vi "Update State.vi"(8 "error in (no error)":errorcluster, 11 "Elevator Controller in":refnum<class "Elevator Controller.lvclass">) -> (0 "error out":errorcluster, 3 "Elevator Controller out":refnum<class "Elevator Controller.lvclass">)   [LabVIEW 2022 SP3, in "Elevator Controller.lvlib" / "Elevator Controller.lvclass"]
uses:
  Elevator Controller.lvclass
  Sim User Console Actor/Abstract User Console Actor/Sim User Console Actor.lvclass
  Abstract User Console Actor/Abstract User Console Actor/Elevator Call.ctl
  Abstract User Console Actor/Abstract User Console Actor/Abstract User Console Actor.lvclass
  Abstract User Console Actor/Abstract User Console Actor/Floor Selection.ctl
  Sim Display Console Actor/Sim Display Console Actor/Sim Display Console Actor.lvclass
  Sim Sensor Interface Actor/Sim Sensor Interface Actor/Sim Sensor Interface Actor.lvclass
  States -Enum.ctl
  Configuration Database Actor/Configuration Database Actor/Configuration Database Actor.lvclass
  <vilib>/ActorFramework/Actor/Actor.lvclass
  Incoming Messages/Set State Msg/Set State Msg.lvclass
  C:/Program Files/National Instruments/LabVIEW 2022/vi.lib/ActorFramework/Actor/Actor.lvclass
  C:/Workspace/CLA/Elevator AF_2022/Elevator Controller/Elevator Controller/Elevator Controller.lvclass
  C:/Workspace/CLA/Elevator AF_2022/Incoming/Incoming.lvclass
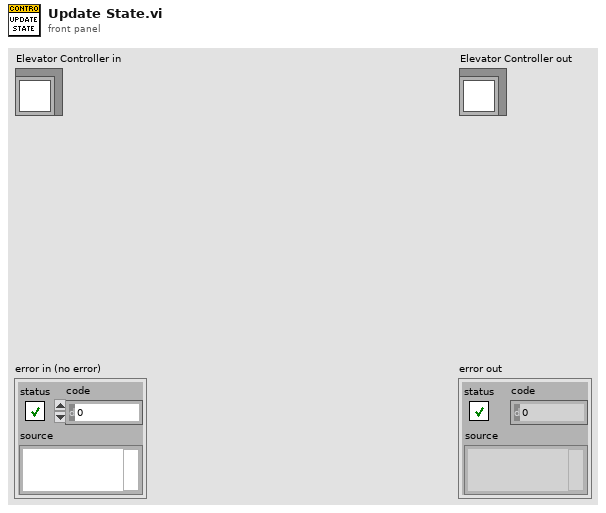
[diagram p1: front panel]
types:
  T1 = typedef "Abstract User Console Actor.lvlib/Abstract User Console Actor.lvclass/Floor Selection.ctl" = cluster{"Floor4":bool, "Floor 3":bool, "Floor2":bool, "Floor1":bool}
  T2 = typedef "Abstract User Console Actor.lvlib/Abstract User Console Actor.lvclass/Elevator Call.ctl" = cluster{"Up":bool, "Up 2":bool, "Up 3":bool, "Down":bool, "Down 2":bool, "Down 3":bool}
  T3 = typedef "Elevator Controller.lvlib/Elevator Controller.lvclass/States -Enum.ctl" = enum16{"Initial State", "Wait for First Request", "Start and Move State", "Analysis State", "Continue Travel State", "Stop at Floor", "Open and Close Door Sequence", "No Request Remaining", "Emergency Call", "Terminate Process", ""}
  T4 = enum8{"Enabled", "Disabled", "Disabled and Grayed Out"}
  T5 = typedef "Configuration Database Actor.lvlib/Configuration Database Actor.lvclass/Time Table.ctl" = cluster{"Open Door":u32, "Close Door":u32, "Travel Time":u32, "Inactivity Time":u32}
  T6 = typedef "Abstract User Console Actor.lvlib/Abstract User Console Actor.lvclass/Door Buttons.ctl" = cluster{"Open Door":bool, "Close Door":bool}
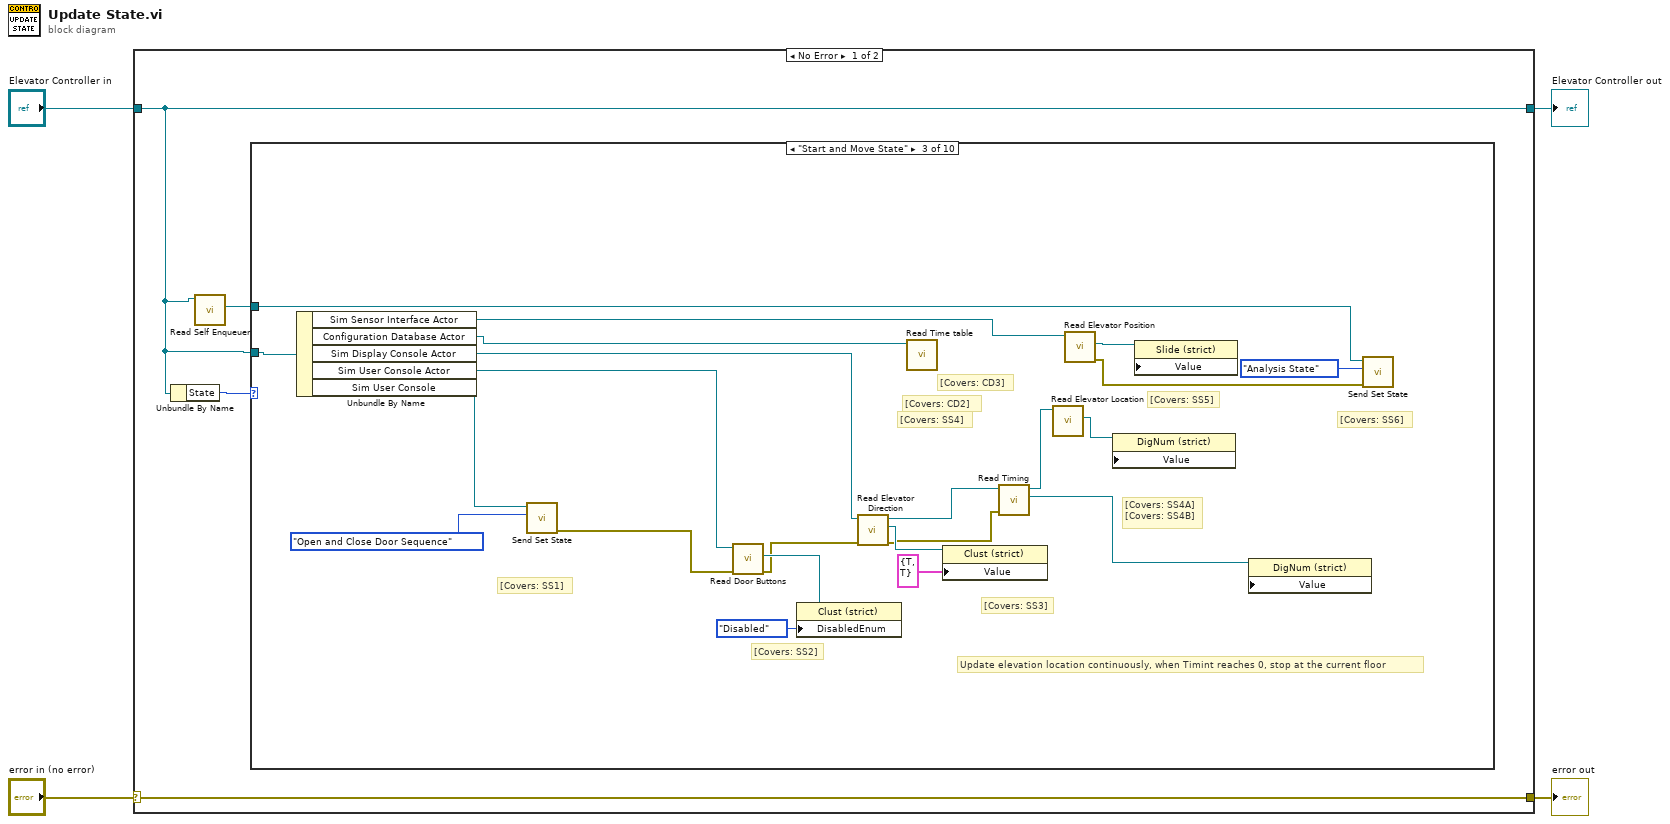
[diagram p0: block diagram]
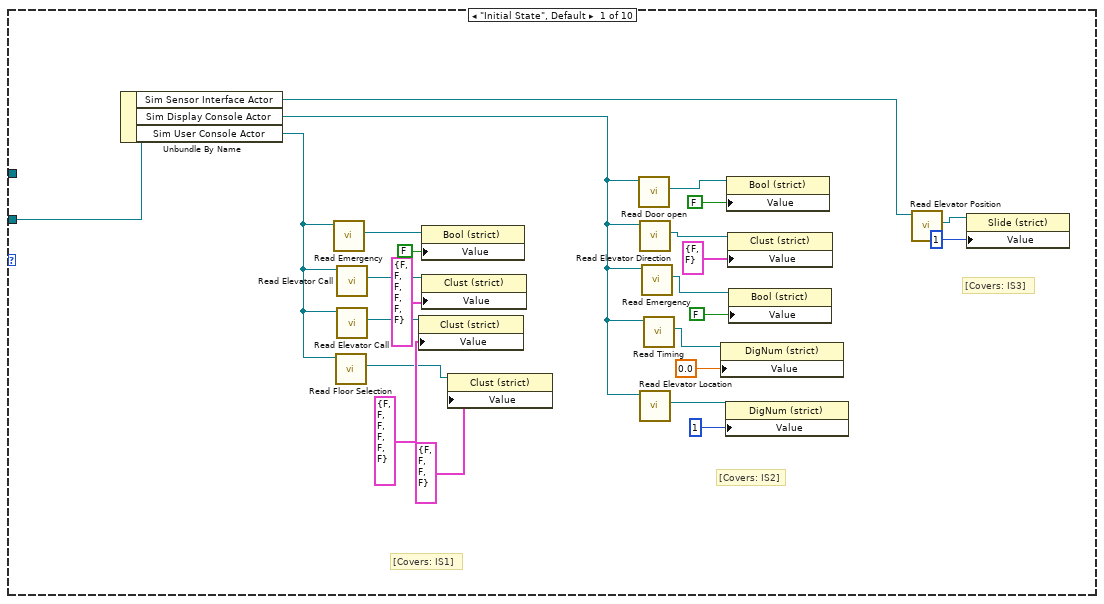
[diagram p2: hidden frame]
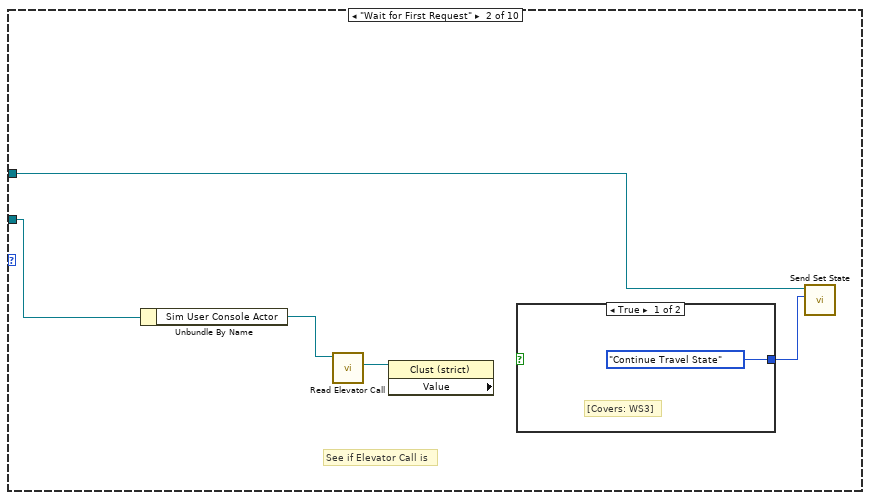
[diagram p3: hidden frame]
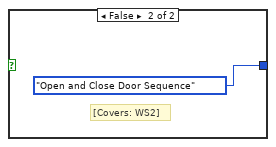
[diagram p4: hidden frame]
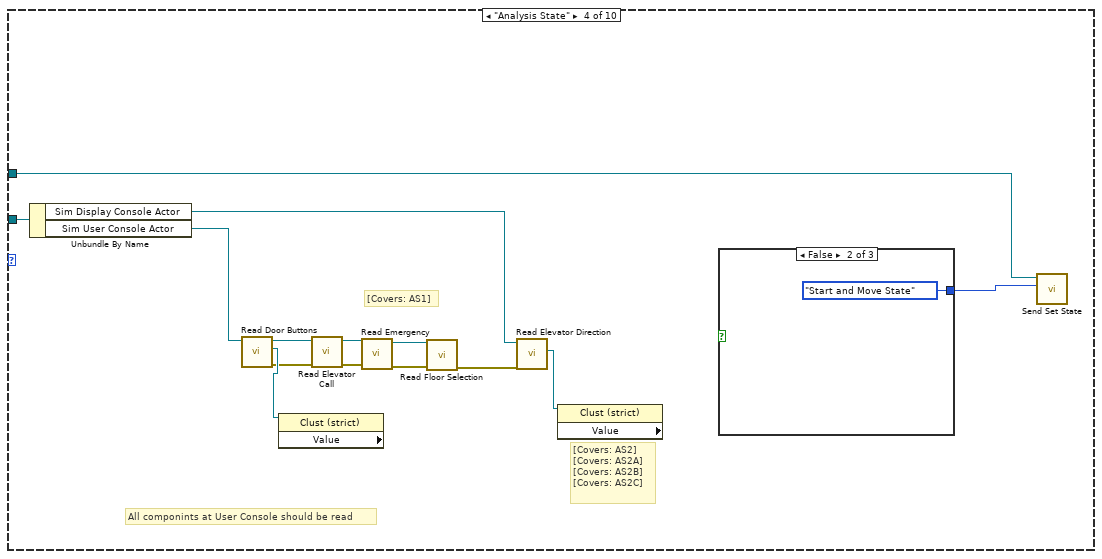
[diagram p5: hidden frame]
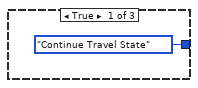
[diagram p6: hidden frame]
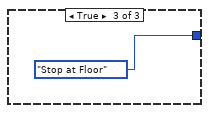
[diagram p7: hidden frame]
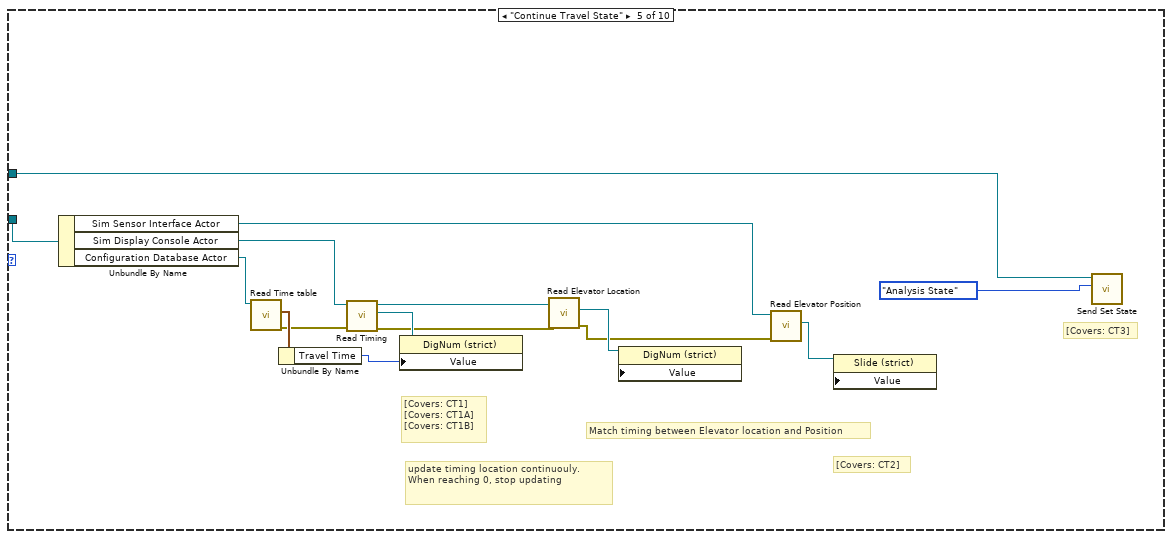
[diagram p8: hidden frame]
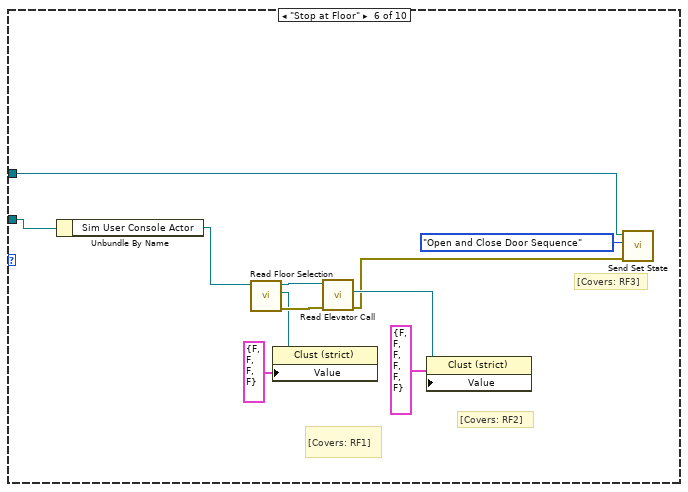
[diagram p9: hidden frame]
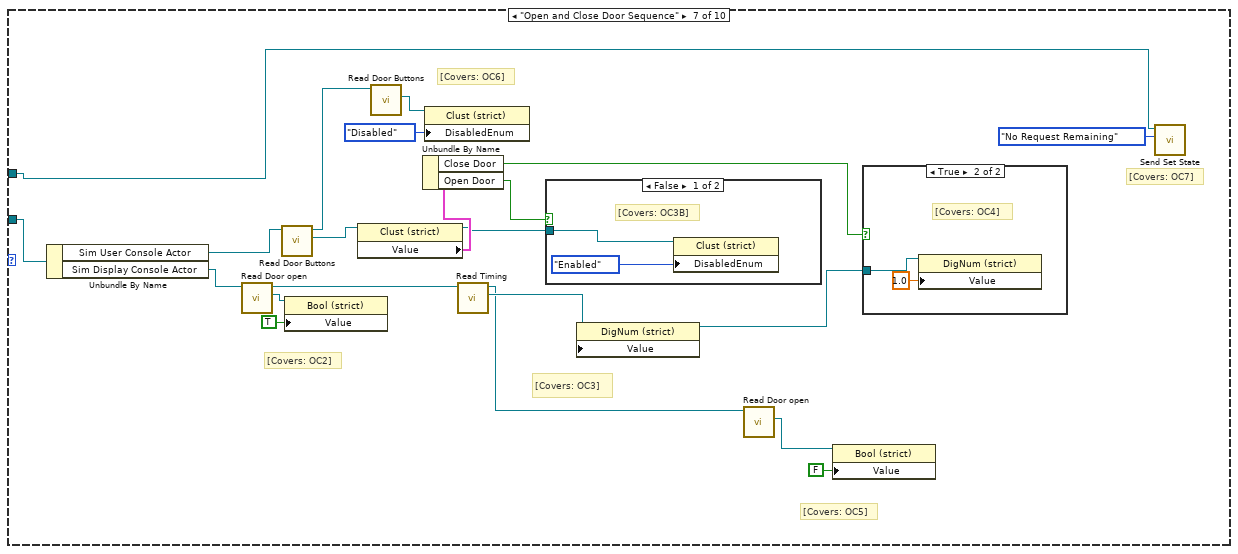
[diagram p10: hidden frame]
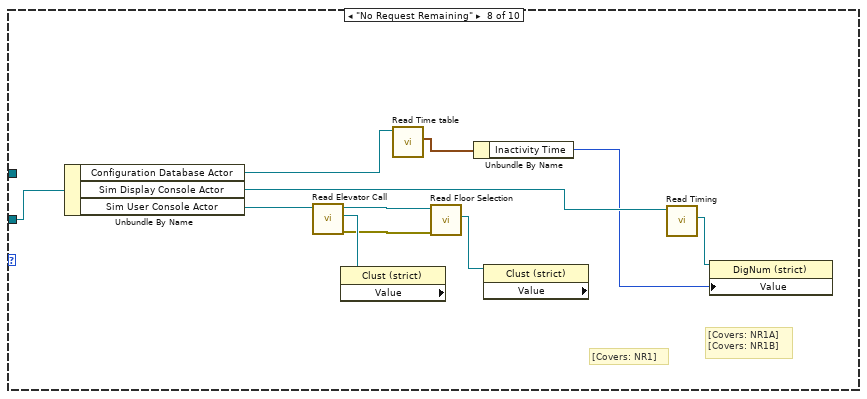
[diagram p13: hidden frame]
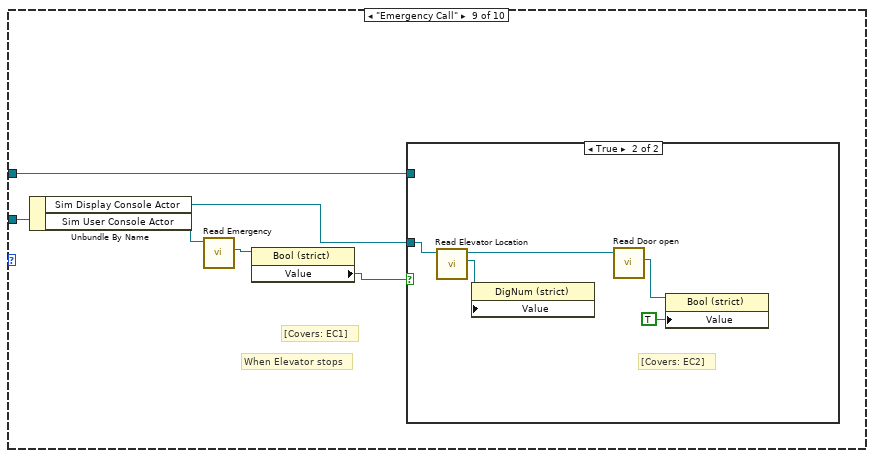
[diagram p14: hidden frame]
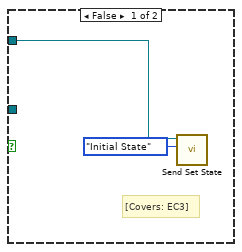
[diagram p15: hidden frame]
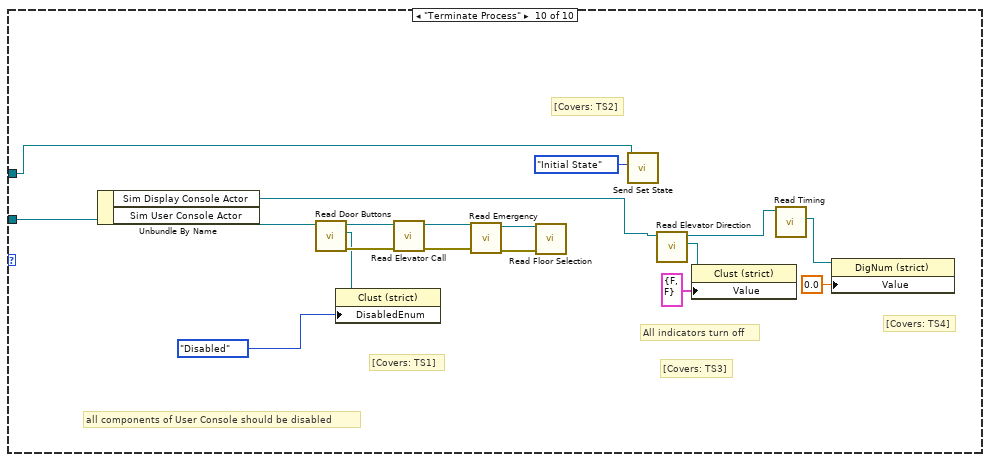
[diagram p16: hidden frame]
diagram:
  n1 = case shown="No Error" "error in (no error)" {
    selector: "error in (no error)" -> [w8 w173]
    tunnel: [w8 w173] -> w3
    tunnel: [w6 w172] -> w1
    tunnel: "Elevator Controller in" -> [w6 w172]
    frame No Error {
      n2 = Unbundle By Name(w6) -> ("State"=w7:T3)
      n3 = call <vilib>:"Read Self Enqueuer.vi"("Actor"=w6) -> ("Self Enqueuer"=w5:refnum<class "Message Enqueuer.lvclass">)  [unwired: 10 in]
      n4 = case shown="\"Start and Move State\"" w7 {
        tunnel: w6 -> [w32 w35 w61 w72 w93 w104 w125 w140 w146 w171]
        tunnel: w5 -> [_ w33 w43 w63 w79 w96 w105 _ w141 w160]
        frame "Initial State", Default {
          # "[Covers: IS3]"
          # "[Covers: IS2]"
          # "[Covers: IS1]"
          n5 = Unbundle By Name(w32) -> ("Sim Sensor Interface Actor"=w11:refnum<class "Sim Sensor Interface Actor.lvclass">, "Sim Display Console Actor"=w14:refnum<class "Sim Display Console Actor.lvclass">, "Sim User Console Actor"=w29:refnum<class "Sim User Console Actor.lvclass">)
          n6 = call "Read Emergency.vi"("Sim User Console Actor in"=w29) -> ("Emergency"=w28:refnum<vi>)  [unwired: 8 in, 2 out]
          n7 = call "Read Floor Selection.vi"("Sim User Console Actor in"=w29) -> ("Floor Selection"=w24:refnum<vi>)  [unwired: 8 in, 2 out]
          n8 = call "Read Elevator Call.vi"("Sim User Console Actor in"=w29) -> ("Elevator Call"=w26:refnum<vi>)  [unwired: 8 in, 2 out]
          n9 = call "Read Elevator Call.vi"("Sim User Console Actor in"=w29) -> ("Elevator Call"=w31:refnum<vi>)  [unwired: 8 in, 2 out]
          n10 = property class="Clust (strict)"(reference=w31, "Value"=T2 {"Up"=FALSE, "Up 2"=FALSE, "Up 3"=FALSE, "Down"=FALSE, "Down 2"=FALSE, "Down 3"=FALSE}) -> ()  [unwired: 1 in, 2 out]
          n11 = property class="Bool (strict)"(reference=w28, "Value"=FALSE) -> ()  [unwired: 1 in, 2 out]
          n12 = property class="Clust (strict)"(reference=w26, "Value"=T2 {"Up"=FALSE, "Up 2"=FALSE, "Up 3"=FALSE, "Down"=FALSE, "Down 2"=FALSE, "Down 3"=FALSE}) -> ()  [unwired: 1 in, 2 out]
          n13 = property class="Clust (strict)"(reference=w24, "Value"=T1 {"Floor4"=FALSE, "Floor 3"=FALSE, "Floor2"=FALSE, "Floor1"=FALSE}) -> ()  [unwired: 1 in, 2 out]
          n14 = call "Read Door open.vi"("Sim Display Console Actor in"=w14) -> ("Door open"=w22:refnum<vi>)  [unwired: 8 in, 2 out]
          n15 = call "Read Elevator Direction.vi"("Sim Display Console Actor in"=w14) -> ("Elevator Direction"=w20:refnum<vi>)  [unwired: 8 in, 2 out]
          n16 = call "Read Elevator Location.vi"("Sim Display Console Actor in"=w14) -> ("Elevator Location"=w13:refnum<vi>)  [unwired: 8 in, 2 out]
          n17 = call "Read Emergency.vi"("Sim Display Console Actor in"=w14) -> ("Emergency"=w18:refnum<vi>)  [unwired: 8 in, 2 out]
          n18 = call "Read Timing.vi"("Sim Display Console Actor in"=w14) -> ("Timing"=w16:refnum<vi>)  [unwired: 8 in, 2 out]
          n19 = property class="DigNum (strict)"(reference=w16, "Value"=0.0) -> ()  [unwired: 1 in, 2 out]
          n20 = property class="DigNum (strict)"(reference=w13, "Value"=u32 1) -> ()  [unwired: 1 in, 2 out]
          n21 = property class="Bool (strict)"(reference=w22, "Value"=FALSE) -> ()  [unwired: 1 in, 2 out]
          n22 = property class="Clust (strict)"(reference=w20, "Value"=cluster{"Up":bool, "Down":bool} {"Up"=FALSE, "Down"=FALSE}) -> ()  [unwired: 1 in, 2 out]
          n23 = property class="Bool (strict)"(reference=w18, "Value"=FALSE) -> ()  [unwired: 1 in, 2 out]
          n24 = call "Read Elevator Position.vi"("Sim Sensor Interface Actor in"=w11) -> ("Elevator Position"=w10:refnum<vi>)  [unwired: 8 in, 2 out]
          n25 = property class="Slide (strict)"(reference=w10, "Value"=u32 1) -> ()  [unwired: 1 in, 2 out]
        }
        frame "Wait for First Request" {
          # "See if Elevator Call is"
          n26 = Unbundle By Name(w35) -> ("Sim User Console Actor"=w37:refnum<class "Sim User Console Actor.lvclass">)
          n27 = call "Read Elevator Call.vi"("Sim User Console Actor in"=w37) -> ("Elevator Call"=w36:refnum<vi>)  [unwired: 8 in, 2 out]
          n28 = property class="Clust (strict)" props=["Value"](reference=w36) -> ()  [unwired: 1 in, 3 out]
          n29 = case shown="\"another call\"" {
            selector: _ -> [_ _]
            tunnel: [States_-Enum."Continue Travel State" ("Enum") States_-Enum."Open and Close Door Sequence" ("Enum")] -> w34
            frame True {
              # "[Covers: WS3]"
            }
            frame False {
              # "[Covers: WS2]"
            }
          }
          n30 = call "Send Set State.vi"("State"=w34, "Message Enqueuer"=w33) -> ()  [unwired: 8 in, 2 out]
        }
        frame "Start and Move State" {
          # "[Covers: CD3]"
          # "[Covers: SS6]"
          # "[Covers: SS5]"
          # "[Covers: CD2]"
          # "[Covers: SS4]"
          # "[Covers: SS4A]\n[Covers: SS4B]"
          # "Update elevation location continuously, when Timint reaches 0, stop at the current floor"
          # "[Covers: SS3]"
          # "[Covers: SS1]"
          # "[Covers: SS2]"
          n31 = Unbundle By Name(w61) -> ("Sim Sensor Interface Actor"=w45:refnum<class "Sim Sensor Interface Actor.lvclass">, "Configuration Database Actor"=w46:refnum<class "Configuration Database Actor.lvclass">, "Sim Display Console Actor"=w54:refnum<class "Sim Display Console Actor.lvclass">, "Sim User Console Actor"=w60:refnum<class "Sim User Console Actor.lvclass">, "Sim User Console"=w57:refnum<class "Message Enqueuer.lvclass">)
          n32 = call "Send Set State.vi"("State"=States_-Enum."Open and Close Door Sequence" ("Enum"), "Message Enqueuer"=w57) -> ("error out"=w55:errorcluster)  [unwired: 8 in, 1 out]
          n33 = call "Read Door Buttons.vi"("error in (no error)"=w55, "Sim User Console Actor in"=w60) -> ("error out"=w53:errorcluster, "Door Buttons"=w59:refnum<vi>)  [unwired: 7 in, 1 out]
          n34 = property class="Clust (strict)"(reference=w59, "DisabledEnum"=T4."Disabled" ("Disabled")) -> ()  [unwired: 1 in, 2 out]
          n35 = call "Read Elevator Direction.vi"("error in (no error)"=w53, "Sim Display Console Actor in"=w54) -> ("error out"=w41:errorcluster, "Elevator Direction"=w52:refnum<vi>, "Sim Display Console Actor out"=w50:refnum<class "Sim Display Console Actor.lvclass">)  [unwired: 7 in]
          n36 = call "Read Time table.vi"("Configuration Database Actor in"=w46) -> ()  [unwired: 8 in, 3 out]
          n37 = property class="Clust (strict)"(reference=w52, "Value"=cluster{"Up":bool, "Down":bool} {"Up"=TRUE, "Down"=TRUE}) -> ()  [unwired: 1 in, 2 out]
          n38 = call "Read Timing.vi"("error in (no error)"=w41, "Sim Display Console Actor in"=w50) -> ("Timing"=w49:refnum<vi>, "Sim Display Console Actor out"=w48:refnum<class "Sim Display Console Actor.lvclass">)  [unwired: 7 in, 1 out]
          n39 = call "Read Elevator Location.vi"("Sim Display Console Actor in"=w48) -> ("Elevator Location"=w47:refnum<vi>)  [unwired: 8 in, 2 out]
          n40 = call "Read Elevator Position.vi"("Sim Sensor Interface Actor in"=w45) -> ("error out"=w40:errorcluster, "Elevator Position"=w44:refnum<vi>)  [unwired: 8 in, 1 out]
          n41 = property class="DigNum (strict)" props=["Value"](reference=w47) -> ()  [unwired: 2 in, 2 out]
          n42 = property class="Slide (strict)" props=["Value"](reference=w44) -> ()  [unwired: 2 in, 2 out]
          n43 = property class="DigNum (strict)" props=["Value"](reference=w49) -> ()  [unwired: 2 in, 2 out]
          n44 = call "Send Set State.vi"("error in (no error)"=w40, "State"=States_-Enum."Analysis State" ("Enum"), "Message Enqueuer"=w43) -> ()  [unwired: 7 in, 2 out]
        }
        frame "Analysis State" {
          # "[Covers: AS2] \n[Covers: AS2A] \n[Covers: AS2B] \n[Covers: AS2C]"
          # "[Covers: AS1]"
          # "All componints at User Console should be read"
          n45 = Unbundle By Name(w72) -> ("Sim Display Console Actor"=w70:refnum<class "Sim Display Console Actor.lvclass">, "Sim User Console Actor"=w71:refnum<class "Sim User Console Actor.lvclass">)
          n46 = call "Read Door Buttons.vi"("Sim User Console Actor in"=w71) -> ("error out"=w68:errorcluster, "Door Buttons"=w69:refnum<vi>, "Sim User Console Actor out"=w75:refnum<class "Sim User Console Actor.lvclass">)  [unwired: 8 in]
          n47 = property class="Clust (strict)" props=["Value"](reference=w69) -> ()  [unwired: 1 in, 3 out]
          n48 = call "Read Elevator Call.vi"("error in (no error)"=w68, "Sim User Console Actor in"=w75) -> ("error out"=w67:errorcluster, "Sim User Console Actor out"=w74:refnum<class "Sim User Console Actor.lvclass">)  [unwired: 7 in, 1 out]
          n49 = call "Read Emergency.vi"("error in (no error)"=w67, "Sim User Console Actor in"=w74) -> ("error out"=w66:errorcluster, "Sim User Console Actor out"=w73:refnum<class "Sim User Console Actor.lvclass">)  [unwired: 7 in, 1 out]
          n50 = call "Read Floor Selection.vi"("error in (no error)"=w66, "Sim User Console Actor in"=w73) -> ("error out"=w65:errorcluster)  [unwired: 7 in, 2 out]
          n51 = call "Read Elevator Direction.vi"("error in (no error)"=w65, "Sim Display Console Actor in"=w70) -> ("Elevator Direction"=w64:refnum<vi>)  [unwired: 7 in, 2 out]
          n52 = property class="Clust (strict)" props=["Value"](reference=w64) -> ()  [unwired: 1 in, 3 out]
          n53 = case shown="\"Change Direction\"" {
            selector: _ -> [_ _ _]
            tunnel: [States_-Enum."Continue Travel State" ("Enum") States_-Enum."Start and Move State" ("Enum") States_-Enum."Stop at Floor" ("Enum")] -> w62
            frame True {
            }
            frame False {
            }
            frame True {
            }
          }
          n54 = call "Send Set State.vi"("State"=w62, "Message Enqueuer"=w63) -> ()  [unwired: 8 in, 2 out]
        }
        frame "Continue Travel State" {
          # "[Covers: CT3]"
          # "Match timing between Elevator location and Position"
          # "[Covers: CT2]"
          # "update timing location continuouly.\nWhen reaching 0, stop updating"
          # "[Covers: CT1] \n[Covers: CT1A] \n[Covers: CT1B]"
          n55 = Unbundle By Name(w93) -> ("Sim Sensor Interface Actor"=w83:refnum<class "Sim Sensor Interface Actor.lvclass">, "Sim Display Console Actor"=w91:refnum<class "Sim Display Console Actor.lvclass">, "Configuration Database Actor"=w92:refnum<class "Configuration Database Actor.lvclass">)
          n56 = call "Read Time table.vi"("Configuration Database Actor in"=w92) -> ("error out"=w86:errorcluster, "Time table (Second)"=w89:T5)  [unwired: 8 in, 1 out]
          n57 = Unbundle By Name(w89) -> ("Travel Time"=w88:u32)
          n58 = call "Read Timing.vi"("error in (no error)"=w86, "Sim Display Console Actor in"=w91) -> ("error out"=w85:errorcluster, "Timing"=w90:refnum<vi>, "Sim Display Console Actor out"=w87:refnum<class "Sim Display Console Actor.lvclass">)  [unwired: 7 in]
          n59 = property class="DigNum (strict)"(reference=w90, "Value"=w88) -> ()  [unwired: 1 in, 2 out]
          n60 = call "Read Elevator Location.vi"("error in (no error)"=w85, "Sim Display Console Actor in"=w87) -> ("error out"=w82:errorcluster, "Elevator Location"=w84:refnum<vi>)  [unwired: 7 in, 1 out]
          n61 = property class="DigNum (strict)" props=["Value"](reference=w84) -> ()  [unwired: 2 in, 2 out]
          n62 = call "Read Elevator Position.vi"("error in (no error)"=w82, "Sim Sensor Interface Actor in"=w83) -> ("Elevator Position"=w81:refnum<vi>)  [unwired: 7 in, 2 out]
          n63 = property class="Slide (strict)" props=["Value"](reference=w81) -> ()  [unwired: 2 in, 2 out]
          n64 = call "Send Set State.vi"("State"=States_-Enum."Analysis State" ("Enum"), "Message Enqueuer"=w79) -> ()  [unwired: 8 in, 2 out]
        }
        frame "Stop at Floor" {
          # "[Covers: RF3]"
          # "[Covers: RF2]"
          # "[Covers: RF1]"
          n65 = Unbundle By Name(w104) -> ("Sim User Console Actor"=w101:refnum<class "Sim User Console Actor.lvclass">)
          n66 = call "Read Floor Selection.vi"("Sim User Console Actor in"=w101) -> ("error out"=w102:errorcluster, "Floor Selection"=w100:refnum<vi>, "Sim User Console Actor out"=w103:refnum<class "Sim User Console Actor.lvclass">)  [unwired: 8 in]
          n67 = property class="Clust (strict)"(reference=w100, "Value"=T1 {"Floor4"=FALSE, "Floor 3"=FALSE, "Floor2"=FALSE, "Floor1"=FALSE}) -> ()  [unwired: 1 in, 2 out]
          n68 = call "Read Elevator Call.vi"("error in (no error)"=w102, "Sim User Console Actor in"=w103) -> ("error out"=w94:errorcluster, "Elevator Call"=w98:refnum<vi>)  [unwired: 7 in, 1 out]
          n69 = property class="Clust (strict)"(reference=w98, "Value"=T2 {"Up"=FALSE, "Up 2"=FALSE, "Up 3"=FALSE, "Down"=FALSE, "Down 2"=FALSE, "Down 3"=FALSE}) -> ()  [unwired: 1 in, 2 out]
          n70 = call "Send Set State.vi"("error in (no error)"=w94, "State"=States_-Enum."Open and Close Door Sequence" ("Enum"), "Message Enqueuer"=w96) -> ()  [unwired: 7 in, 2 out]
        }
        frame "Open and Close Door Sequence" {
          # "[Covers: OC7]"
          # "[Covers: OC6]"
          # "[Covers: OC5]"
          # "[Covers: OC3]"
          # "[Covers: OC2]"
          n71 = Unbundle By Name(w125) -> ("Sim User Console Actor"=w119:refnum<class "Sim User Console Actor.lvclass">, "Sim Display Console Actor"=w124:refnum<class "Sim Display Console Actor.lvclass">)
          n72 = call "Read Door open.vi"("Sim Display Console Actor in"=w124) -> ("Door open"=w123:refnum<vi>, "Sim Display Console Actor out"=w121:refnum<class "Sim Display Console Actor.lvclass">)  [unwired: 8 in, 1 out]
          n73 = call "Read Door Buttons.vi"("Sim User Console Actor in"=w119) -> ("Door Buttons"=w118:refnum<vi>, "Sim User Console Actor out"=w109:refnum<class "Sim User Console Actor.lvclass">)  [unwired: 8 in, 1 out]
          n74 = property class="Bool (strict)"(reference=w123, "Value"=TRUE) -> ()  [unwired: 1 in, 2 out]
          n75 = property class="Clust (strict)"(reference=w118) -> (reference out=w115:refnum<vi>, "Value"=w117:T6)  [unwired: 1 in, 1 out]
          n76 = call "Read Door Buttons.vi"("Sim User Console Actor in"=w109) -> ("Door Buttons"=w108:refnum<vi>)  [unwired: 8 in, 2 out]
          n77 = Unbundle By Name(w117) -> ("Close Door"=w114:bool, "Open Door"=w116:bool)
          n78 = property class="Clust (strict)"(reference=w108, "DisabledEnum"=T4."Disabled" ("Disabled")) -> ()  [unwired: 1 in, 2 out]
          n79 = call "Read Timing.vi"("Sim Display Console Actor in"=w121) -> ("Timing"=w120:refnum<vi>, "Sim Display Console Actor out"=w112:refnum<class "Sim Display Console Actor.lvclass">)  [unwired: 8 in, 1 out]
          n80 = case shown="False" w116 {
            tunnel: w115 -> [w129 _]
            frame False {
              # "[Covers: OC3B]"
              n81 = property class="Clust (strict)"(reference=w129, "DisabledEnum"=T4."Enabled" ("Disabled")) -> ()  [unwired: 1 in, 2 out]
            }
            frame True {
              # "[Covers: OC3A]"
            }
          }
          n82 = property class="DigNum (strict)" props=["Value"](reference=w120) -> (reference out=w113:refnum<vi>)  [unwired: 2 in, 1 out]
          n83 = call "Read Door open.vi"("Sim Display Console Actor in"=w112) -> ("Door open"=w111:refnum<vi>)  [unwired: 8 in, 2 out]
          n84 = property class="Bool (strict)"(reference=w111, "Value"=FALSE) -> ()  [unwired: 1 in, 2 out]
          n85 = case shown="True" w114 {
            tunnel: w113 -> [_ w127]
            frame False {
            }
            frame True {
              # "[Covers: OC4]"
              n86 = property class="DigNum (strict)"(reference=w127, "Value"=1.0) -> ()  [unwired: 1 in, 2 out]
            }
          }
          n87 = call "Send Set State.vi"("State"=States_-Enum."No Request Remaining" ("Enum"), "Message Enqueuer"=w105) -> ()  [unwired: 8 in, 2 out]
        }
        frame "No Request Remaining" {
          # "[Covers: NR1A] \n[Covers: NR1B]"
          # "[Covers: NR1]"
          n88 = Unbundle By Name(w140) -> ("Configuration Database Actor"=w132:refnum<class "Configuration Database Actor.lvclass">, "Sim Display Console Actor"=w134:refnum<class "Sim Display Console Actor.lvclass">, "Sim User Console Actor"=w139:refnum<class "Sim User Console Actor.lvclass">)
          n89 = call "Read Elevator Call.vi"("Sim User Console Actor in"=w139) -> ("error out"=w136:errorcluster, "Elevator Call"=w137:refnum<vi>, "Sim User Console Actor out"=w138:refnum<class "Sim User Console Actor.lvclass">)  [unwired: 8 in]
          n90 = property class="Clust (strict)" props=["Value"](reference=w137) -> ()  [unwired: 1 in, 3 out]
          n91 = call "Read Time table.vi"("Configuration Database Actor in"=w132) -> ("Time table (Second)"=w131:T5)  [unwired: 8 in, 2 out]
          n92 = call "Read Floor Selection.vi"("error in (no error)"=w136, "Sim User Console Actor in"=w138) -> ("Floor Selection"=w135:refnum<vi>)  [unwired: 7 in, 2 out]
          n93 = Unbundle By Name(w131) -> ("Inactivity Time"=w130:u32)
          n94 = property class="Clust (strict)" props=["Value"](reference=w135) -> ()  [unwired: 1 in, 3 out]
          n95 = call "Read Timing.vi"("Sim Display Console Actor in"=w134) -> ("Timing"=w133:refnum<vi>)  [unwired: 8 in, 2 out]
          n96 = property class="DigNum (strict)"(reference=w133, "Value"=w130) -> ()  [unwired: 1 in, 2 out]
        }
        frame "Emergency Call" {
          # "When Elevator stops"
          # "[Covers: EC1]"
          n97 = Unbundle By Name(w146) -> ("Sim Display Console Actor"=w142:refnum<class "Sim Display Console Actor.lvclass">, "Sim User Console Actor"=w145:refnum<class "Sim User Console Actor.lvclass">)
          n98 = call "Read Emergency.vi"("Sim User Console Actor in"=w145) -> ("Emergency"=w144:refnum<vi>)  [unwired: 8 in, 2 out]
          n99 = property class="Bool (strict)"(reference=w144) -> ("Value"=w143:bool)  [unwired: 1 in, 2 out]
          n100 = case shown="True" w143 {
            tunnel: w142 -> [_ w153]
            tunnel: w141 -> [w148 _]
            frame False {
              # "[Covers: EC3]"
              n101 = call "Send Set State.vi"("State"=States_-Enum."Initial State" ("Enum"), "Message Enqueuer"=w148) -> ()  [unwired: 8 in, 2 out]
            }
            frame True {
              # "[Covers: EC2]"
              n102 = call "Read Elevator Location.vi"("Sim Display Console Actor in"=w153) -> ("Elevator Location"=w152:refnum<vi>, "Sim Display Console Actor out"=w151:refnum<class "Sim Display Console Actor.lvclass">)  [unwired: 8 in, 1 out]
              n103 = property class="DigNum (strict)" props=["Value"](reference=w152) -> ()  [unwired: 2 in, 2 out]
              n104 = call "Read Door open.vi"("Sim Display Console Actor in"=w151) -> ("Door open"=w150:refnum<vi>)  [unwired: 8 in, 2 out]
              n105 = property class="Bool (strict)"(reference=w150, "Value"=TRUE) -> ()  [unwired: 1 in, 2 out]
            }
          }
        }
        frame "Terminate Process" {
          # "[Covers: TS3]"
          # "[Covers: TS4]"
          # "[Covers: TS2]"
          # "All indicators turn off"
          # "all components of User Console should be disabled"
          # "[Covers: TS1]"
          n106 = Unbundle By Name(w171) -> ("Sim Display Console Actor"=w159:refnum<class "Sim Display Console Actor.lvclass">, "Sim User Console Actor"=w164:refnum<class "Sim User Console Actor.lvclass">)
          n107 = call "Read Door Buttons.vi"("Sim User Console Actor in"=w164) -> ("error out"=w167:errorcluster, "Door Buttons"=w163:refnum<vi>, "Sim User Console Actor out"=w170:refnum<class "Sim User Console Actor.lvclass">)  [unwired: 8 in]
          n108 = property class="Clust (strict)"(reference=w163, "DisabledEnum"=T4."Disabled" ("Disabled")) -> ()  [unwired: 1 in, 2 out]
          n109 = call "Read Elevator Call.vi"("error in (no error)"=w167, "Sim User Console Actor in"=w170) -> ("error out"=w166:errorcluster, "Sim User Console Actor out"=w169:refnum<class "Sim User Console Actor.lvclass">)  [unwired: 7 in, 1 out]
          n110 = call "Read Emergency.vi"("error in (no error)"=w166, "Sim User Console Actor in"=w169) -> ("error out"=w165:errorcluster, "Sim User Console Actor out"=w168:refnum<class "Sim User Console Actor.lvclass">)  [unwired: 7 in, 1 out]
          n111 = call "Read Floor Selection.vi"("error in (no error)"=w165, "Sim User Console Actor in"=w168) -> ()  [unwired: 7 in, 3 out]
          n112 = call "Send Set State.vi"("State"=States_-Enum."Initial State" ("Enum"), "Message Enqueuer"=w160) -> ()  [unwired: 8 in, 2 out]
          n113 = call "Read Elevator Direction.vi"("Sim Display Console Actor in"=w159) -> ("Elevator Direction"=w158:refnum<vi>, "Sim Display Console Actor out"=w156:refnum<class "Sim Display Console Actor.lvclass">)  [unwired: 8 in, 1 out]
          n114 = property class="Clust (strict)"(reference=w158, "Value"=cluster{"Up":bool, "Down":bool} {"Up"=FALSE, "Down"=FALSE}) -> ()  [unwired: 1 in, 2 out]
          n115 = call "Read Timing.vi"("Sim Display Console Actor in"=w156) -> ("Timing"=w155:refnum<vi>)  [unwired: 8 in, 2 out]
          n116 = property class="DigNum (strict)"(reference=w155, "Value"=0.0) -> ()  [unwired: 1 in, 2 out]
        }
      }
    }
    frame Error {
    }
  }
  "error out" <- w3
  "Elevator Controller out" <- w1
